vi "ExSetEMGbl.vi"() -> ()   [LabVIEW 2010]
uses:
  Open-Close Hardware/CamHandle.vi
panel:
  in  "EM setting":dbl=250.0
  out "error out":errorcluster
  in  "error in (no error)":errorcluster
  # "ExSetEMGbl:\nThis sets the EM gain"
  # "NOTICE\n\nTHIS VI USES A GLOBAL CAMERA HANDLE\n\nTHE VI EXOPENGLOBALCAM.VI MUST BE\nRUN AT THE START OF THE WORK SESSION.\nTHE CAMERA WILL REMAIN OPENED.\n\nTHE VI EXCLOSEGLOBALCAM.VI MUST\nBE RUN BEFORE LEAVING LABVIEW."
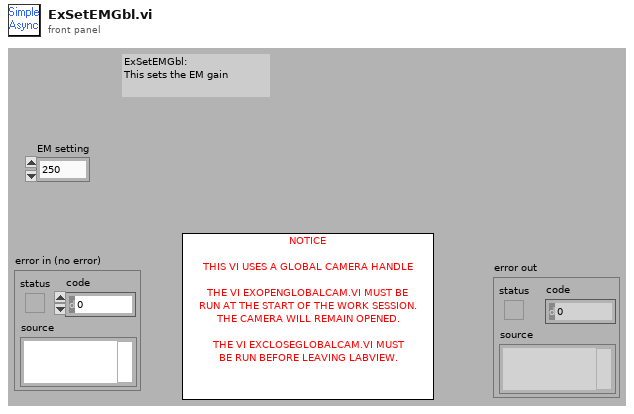
[diagram p1: front panel]
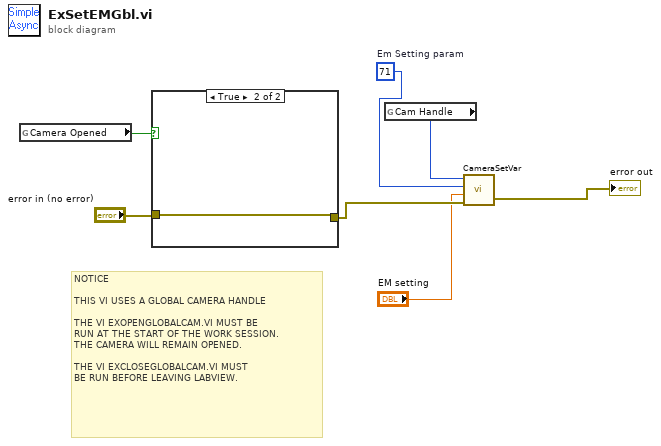
[diagram p0: block diagram]
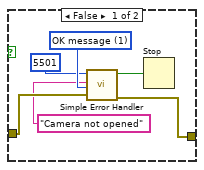
[diagram p2: hidden frame]
diagram:
  w1 = 71  # Em Setting param
  # "NOTICE\n\nTHIS VI USES A GLOBAL CAMERA HANDLE\n\nTHE VI EXOPENGLOBALCAM.VI MUST BE\nRUN AT THE START OF THE WORK SESSION.\nTHE CAMERA WILL REMAIN OPENED.\n\nTHE VI EXCLOSEGLOBALCAM.VI MUST\nBE RUN BEFORE LEAVING LABVIEW."
  n1 = global read "CamHandle.vi" "Camera Opened"() -> (w7:bool)
  n2 = case shown="True" w7 {
    tunnel: "error in (no error)" -> [w12 w14]
    tunnel: [w11 w14] -> w5
    frame False {
      w13 = u16 1 items=["no dialog", "OK message", "continue or stop message"] ("type of dialog (OK msg:1)")
      n3 = call <vilib>:"Simple Error Handler.vi"("error code (no error:0)"=5501, "error source (\" \")"="Camera not opened", "type of dialog (OK msg:1)"=w13, "error in (no error)"=w12) -> ("error?"=w9:bool, "error out"=w11:errorcluster)  [unwired: 1 in, 3 out]
      n4 = Stop(stop? (T)=w9) -> ()
    }
    frame True {
    }
  }
  n5 = global read "CamHandle.vi" "Cam Handle"() -> (w2:u32)
  n6 = call <userlib>:"CameraSetVar.vi"("error in"=w5, "Value"="EM setting", "Parameter ID"=w1, "Camera Handle"=w2) -> ("error out"=→"error out":errorcluster)  [unwired: 1 out]
